vi "GOOP_MyComputer_Item_NotifyChanged.vi"(10 "Change Type":T1=enum."Item Modified", 11 "Object":u64) -> ()   [LabVIEW 2014]
uses:
  <resource>/Framework/Providers/API/mxLvChangeType.ctl
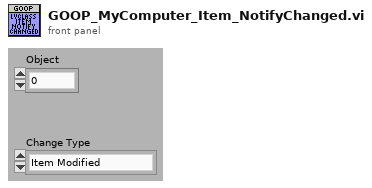
[diagram p1: front panel]
types:
  T1 = typedef "mxLvChangeType.ctl" = enum32{"Item Created", "Item Modified", "File Modified", "File Deleted", "Item Added", "Item Added to SCC", "Item Renamed", "Item Modified For SCC"}
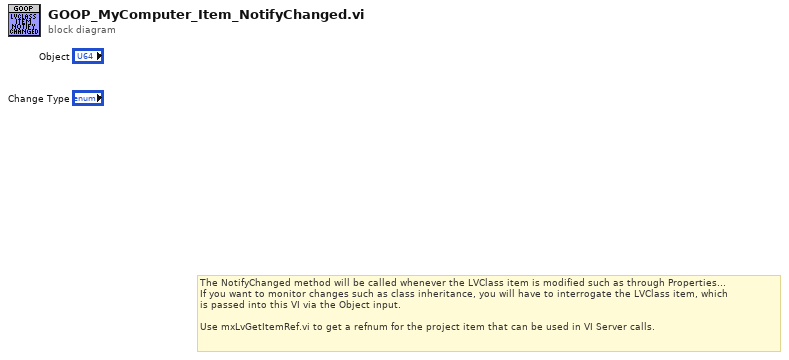
[diagram p0: block diagram]
diagram:
  # "The NotifyChanged method will be called whenever the LVClass item is modified such as through Properties...\nIf you want to monitor changes such as class inheritance, you will have to interrogate the LVClass item, which\nis passed into this VI via the Object input.\n\nUse mxLvGetItemRef.vi to get a refnum for the project item that can be used in VI Server calls."
